vi "Read stored tag set.vi"(8 "error in (no error)":errorcluster, 11 "stored tags":T3[](array[typedef])) -> (0 "error out":errorcluster, 3 "Tags":T1[](array[typedef]))   [LabVIEW 2020, in "Current Value Table(Rebuild).lvlib"]
uses:
  Current Value Table(Rebuild).lvlib
  Type Defs/Data Types.ctl
  Type Defs/Single Tag.ctl
  Type Defs/Tag in Memory.ctl
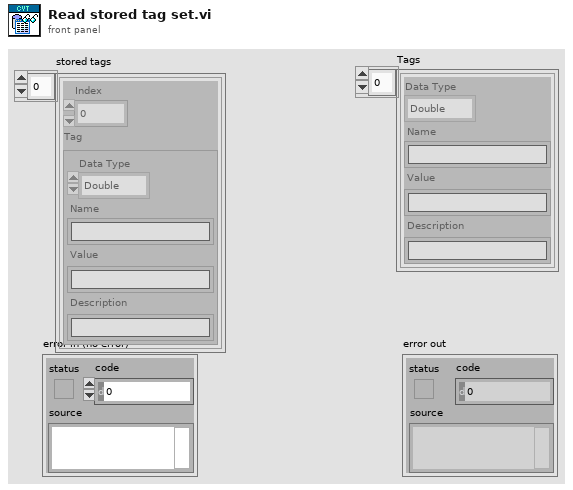
[diagram p1: front panel]
types:
  T1 = typedef "Current Value Table(Rebuild).lvlib/Single Tag.ctl" = cluster{"Data Type":T2, "Name":string, "Value":string, "Description":string}
  T2 = typedef "Current Value Table(Rebuild).lvlib/Data Types.ctl" = enum16{"Double", "Single", "I64", "I32", "I16", "I8", "U64", "U32", "U16", "U8", "String", "Boolean", "Array of U8", "Array of U16", "Array of U32", "Array of U64", "Array of I64", "Array of I32", "Array of I16", "Array of I8", "Array of Double", "Array of Single", "Array of Boolean", "Array of String"}
  T3 = typedef "Current Value Table(Rebuild).lvlib/Tag in Memory.ctl" = cluster{"Index":i32, "Tag":T1}
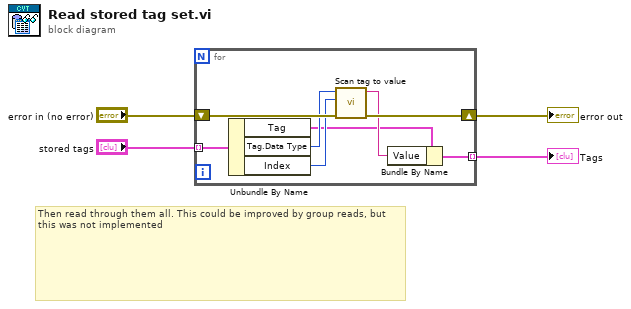
[diagram p0: block diagram]
diagram:
  # "Then read through them all. This could be improved by group reads, but this was not implemented"
  n1 = for {
    shift-right: [w11] -> w2
    shift-left: "error in (no error)" -> [w9]
    tunnel: "stored tags" -> [w12] mode=indexing
    tunnel: [w8] -> w1 mode=indexing
    n2 = Unbundle By Name(w12) -> ("Tag"=w5:T1, "Tag.Data Type"=w7:T2, "Index"=w6:i32)
    n3 = call "Scan tag to value.vi"("error in (no error)"=w9, "Index"=w6, "Data Type"=w7) -> ("error out"=w11:errorcluster, "Value"=w10:string)  [unwired: 7 in]
    n4 = Bundle By Name(cluster=w5, "Value"=w10) -> (w8:T1)
  }
  "error out" <- w2
  "Tags" <- w1
